vi "Sub_KDELTA.vi"(9 "Pin-Location":i32, 10 "Pre-Pin Matrix":dbl[][](array[numeric])) -> (3 "K12":dbl[][](array[numeric]))   [LabVIEW 2019]
uses:
  <vilib>/Analysis/Matrix/Numeric/Conversions/Matrix To Array - RM.vi
  <vilib>/Analysis/Matrix/NI_Matrix.lvlib
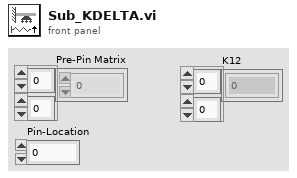
[diagram p1: front panel]
types:
  T1 = typedef "NI_Matrix.lvlib/RealMatrix.ctl" = dbl[][]
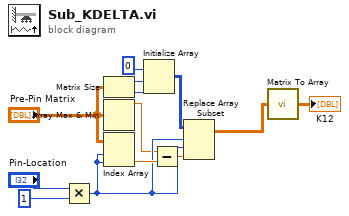
[diagram p0: block diagram]
diagram:
  n1 = Multiply(x="Pin-Location", y=1) -> (x*y=w3:i32)
  n2 = Matrix Size(0:"Pre-Pin Matrix") -> (1:w8:i32, 2:w9:i32)
  n3 = Array Max & Min(array="Pre-Pin Matrix") -> (max value=w1:dbl)  [unwired: 3 out]
  n4 = Index Array(array="Pre-Pin Matrix", index (row)=w3, index (col)=w3) -> (element=w5:dbl)
  n5 = Initialize Array(0, w8, w9) -> (w4:i32[][])
  n6 = Subtract(x=w1, y=w5) -> (x-y=w6:dbl)
  n7 = Replace Array Subset(array=w4, new element=w6, index (row)=w3, index (col)=w3) -> (w12:T1)
  n8 = call-poly <vilib>:"Matrix To Array.vi"("Real Matrix"=w12) -> ("Real 2D Array"=→"K12":dbl[][])
